vi "SSL Detection Frame Simple Estimator.vi"(7 "Enable":bool=TRUE, 10 "Field Size":T1, 11 "Detection Frame In":T2 {"robots_blue"."height" format="%+4.3f"; "robots_blue"."pixel_y" format="%+4.3f"; "robots_blue"."pixel_x" format="%+4.3f"; "robots_blue"."orientation" format="%+4.3f"; "robots_blue"."y" format="%+4.3f"; "robots_blue"."confidence" format="%4.3f"; "robots_blue"."x" format="%+4.3f"; "robots_yellow"."height" format="%+4.3f"; "robots_yellow"."pixel_y" format="%+4.3f"; "robots_yellow"."pixel_x" format="%+4.3f"; "robots_yellow"."orientation" format="%+4.3f"; "robots_yellow"."y" format="%+4.3f"; "robots_yellow"."confidence" format="%4.3f"; "robots_yellow"."x" format="%+4.3f"}) -> (2 "Field Size Out":T1, 3 "Detection Frame Out":T2 {"robots_blue"."height" format="%+4.3f"; "robots_blue"."pixel_y" format="%+4.3f"; "robots_blue"."pixel_x" format="%+4.3f"; "robots_blue"."orientation" format="%+4.3f"; "robots_blue"."y" format="%+4.3f"; "robots_blue"."confidence" format="%4.3f"; "robots_blue"."x" format="%+4.3f"; "robots_yellow"."height" format="%+4.3f"; "robots_yellow"."pixel_y" format="%+4.3f"; "robots_yellow"."pixel_x" format="%+4.3f"; "robots_yellow"."orientation" format="%+4.3f"; "robots_yellow"."y" format="%+4.3f"; "robots_yellow"."confidence" format="%4.3f"; "robots_yellow"."x" format="%+4.3f"})   [LabVIEW 2020]
uses:
  Controls/SSL Detection Frame.ctl
  Controls/SSL Detection Robot.ctl
  <vilib>/Analysis/Matrix/Datatypes/RealMatrix.ctl
  Controls/SSL Detection Ball.ctl
  <vilib>/Analysis/Matrix/NI_Matrix.lvlib
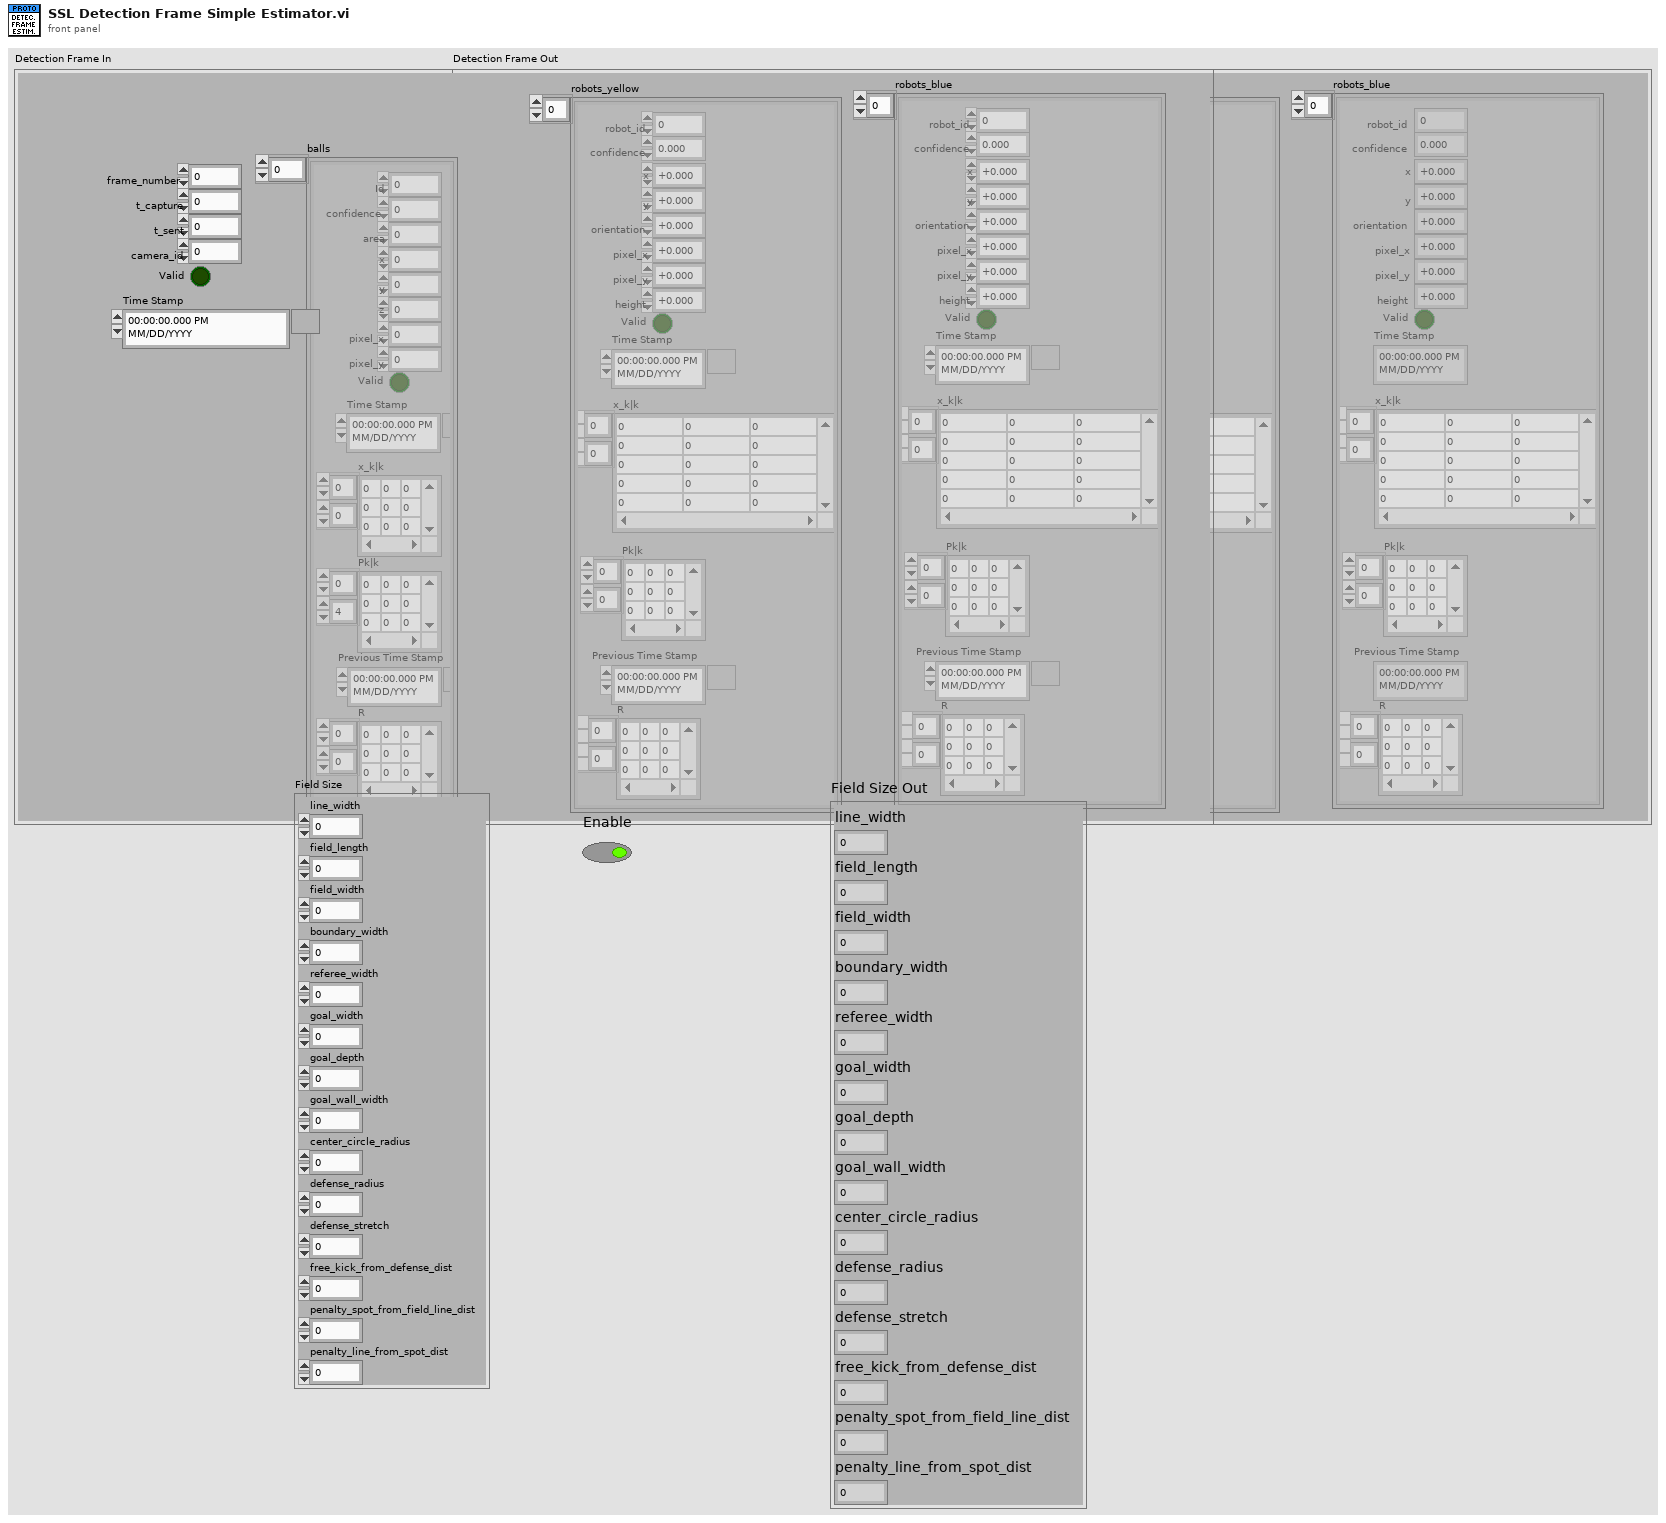
[diagram p1: front panel]
types:
  T1 = cluster{"line_width":u32, "field_length":u32, "field_width":u32, "boundary_width":u32, "referee_width":u32, "goal_width":u32, "goal_depth":u32, "goal_wall_width":u32, "center_circle_radius":u32, "defense_radius":u32, "defense_stretch":u32, "free_kick_from_defense_dist":u32, "penalty_spot_from_field_line_dist":u32, "penalty_line_from_spot_dist":u32}
  T2 = typedef "SSL Detection Frame.ctl" = cluster{"frame_number":u32, "t_capture":dbl, "t_sent":dbl, "camera_id":u32, "robots_yellow":T3[], "robots_blue":T3[], "balls":T5[], "Valid":bool, "Time Stamp":timestamp}
  T3 = typedef "SSL Detection Robot.ctl" = cluster{"x":sgl, "robot_id":u32, "confidence":sgl, "y":sgl, "orientation":sgl, "pixel_x":sgl, "pixel_y":sgl, "height":sgl, "Valid":bool, "Time Stamp":timestamp, "x_k|k":T4, "Pk|k":T4, "Previous Time Stamp":timestamp, "R":T4}
  T4 = typedef "NI_Matrix.lvlib/RealMatrix.ctl" = dbl[][]
  T5 = typedef "SSL Detection Ball.ctl" = cluster{"x":sgl, "area":u32, "confidence":sgl, "y":sgl, "z":sgl, "pixel_x":sgl, "pixel_y":sgl, "Valid":bool, "Time Stamp":timestamp, "x_k|k":T4, "Pk|k":T4, "Id":u32, "Previous Time Stamp":timestamp, "R":T4}
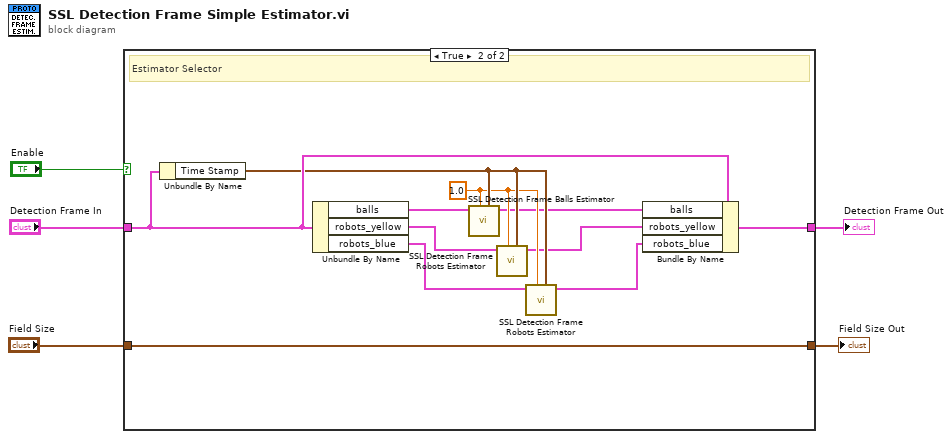
[diagram p0: block diagram]
diagram:
  n1 = case shown="True" "Enable" {
    tunnel: [w7 w18] -> w5
    tunnel: "Detection Frame In" -> [w7 w16]
    tunnel: "Field Size" -> [w6 w17]
    tunnel: [w6 w17] -> w2
    frame False {
    }
    frame True {
      w11 = 1.0 ("Life Time")
      # "Estimator Selector"
      n2 = Unbundle By Name(w16) -> ("Time Stamp"=w15:timestamp)
      n3 = Unbundle By Name(w16) -> ("balls"=w13:T5[], "robots_yellow"=w14:T3[], "robots_blue"=w12:T3[])
      n4 = call "SSL Detection Frame Balls Estimator.vi"("Time Stamp"=w15, "Life Time"=w11, "Balls"=w13) -> ("Est balls"=w8:T5[])  [unwired: 8 in]
      n5 = call "SSL Detection Frame Robots Estimator.vi"("Time Stamp"=w15, "Life Time"=w11, "Robots"=w14) -> ("Est. Robots"=w10:T3[])  [unwired: 8 in]
      n6 = call "SSL Detection Frame Robots Estimator.vi"("Time Stamp"=w15, "Life Time"=w11, "Robots"=w12) -> ("Est. Robots"=w9:T3[])  [unwired: 8 in]
      n7 = Bundle By Name(cluster=w16, "balls"=w8, "robots_yellow"=w10, "robots_blue"=w9) -> (w18:T2)
    }
  }
  "Detection Frame Out" <- w5
  "Field Size Out" <- w2
